vi "CompileFarm_RegistryGUID.vi"() -> ()   [LabVIEW 2011]
panel:
  in  "FarmRegistryKey":string="SOFTWARE\\National Instruments\\NI-Farm\\1.0"
  in  "FarmDll":string="NiFarmClientDll"
  in  "RegistryKey":string="SOFTWARE\\National Instruments\\LabVIEW\\10.0\\AddOns\\LabVIEW for ARM"
  in  "WorkingDirectory":string="WorkingDirectory"
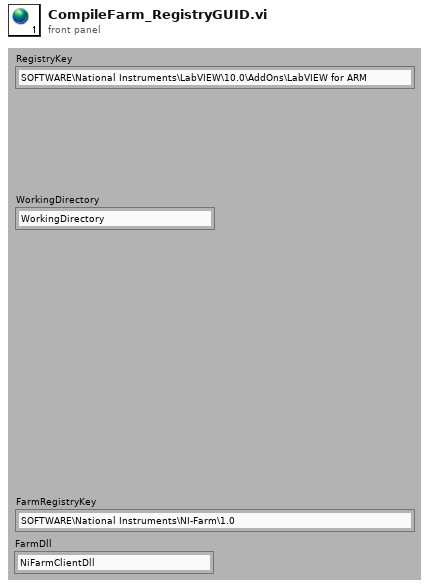
[diagram p1: front panel]
diagram:
